vi "updateEndTime.vi"(8 "error in (no error)":errorcluster, 11 "SingleToneRamp in":refnum<class "SingleToneRamp.lvclass">) -> (0 "error out":errorcluster, 3 "SingleToneRamp out":refnum<class "SingleToneRamp.lvclass">)   [LabVIEW 2011, in "Tools.lvlib" / "Scripting.lvlib" / "SingleToneRamp.lvclass"]
uses:
  SingleToneRamp.lvclass
  SingleToneRamp.lvclass/SingleToneRamp.ctl
  ScriptEvent.lvclass
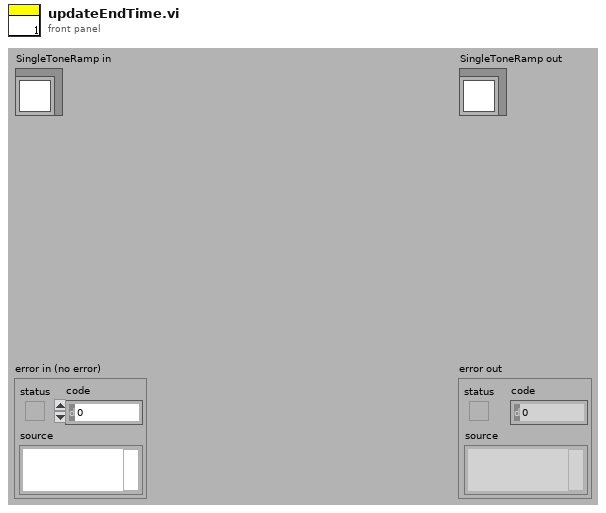
[diagram p1: front panel]
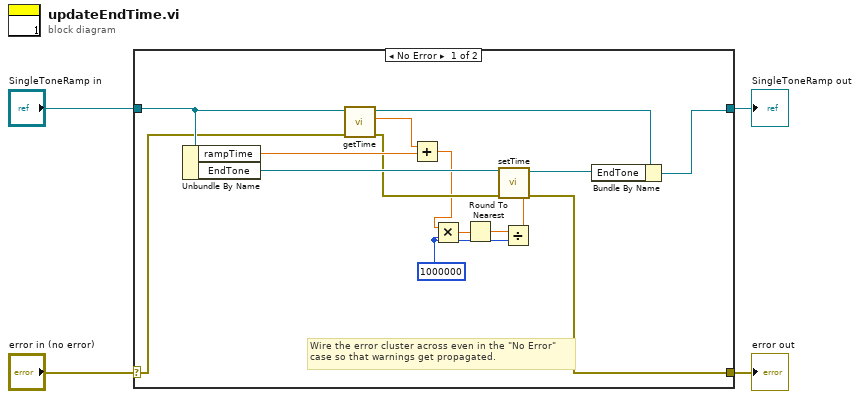
[diagram p0: block diagram]
diagram:
  n1 = case shown="No Error" "error in (no error)" {
    selector: "error in (no error)" -> [w10 w21]
    tunnel: [w12 w21] -> w3
    tunnel: [w13 w20] -> w1
    tunnel: "SingleToneRamp in" -> [w19 w20]
    frame No Error {
      w7 = 1000000
      # "Wire the error cluster across even in the \"No Error\"\ncase so that warnings get propagated."
      n2 = Unbundle By Name(w19) -> ("rampTime"=w17:dbl, "EndTone"=w16:refnum<class "SingleTone.lvclass">)
      n3 = call "getTime.vi"("error in (no error)"=w10, "ScriptEvent.lvclass in"=w19) -> ("error out"=w11:errorcluster, "time"=w18:dbl, "ScriptEvent.lvclass out"=w14:refnum<class "SingleToneRamp.lvclass">)  [unwired: 7 in]
      n4 = Add(x=w18, y=w17) -> (x+y=w6:dbl)
      n5 = Multiply(x=w6, y=w7) -> (x*y=w9:dbl)
      n6 = Round To Nearest(number=w9) -> (nearest integer value=w8:dbl)
      n7 = Divide(x=w8, y=w7) -> (x/y=w5:dbl)
      n8 = call "setTime.vi"("error in (no error)"=w11, "time"=w5, "ScriptEvent.lvclass in"=w16) -> ("error out"=w12:errorcluster, "ScriptEvent.lvclass out"=w15:refnum<class "SingleTone.lvclass">)  [unwired: 7 in]
      n9 = Bundle By Name(cluster=w14, "EndTone"=w15) -> (w13:refnum<class "SingleToneRamp.lvclass">)
    }
    frame Error {
    }
  }
  "error out" <- w3
  "SingleToneRamp out" <- w1
